vi "GetIPAddress.vi"() -> (0 "data out":string)   [LabVIEW 2012]
doc: "Get the RIO's IP address"
panel:
  out "error out":errorcluster
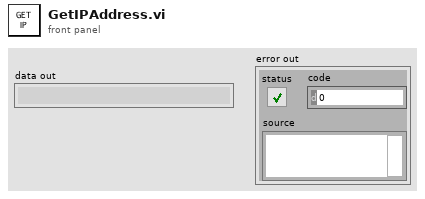
[diagram p1: front panel]
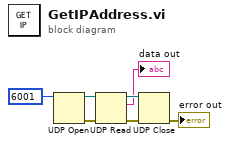
[diagram p0: block diagram]
diagram:
  n1 = UDP Open(11:u16 6001 ("port")) -> (port=w6:refnum<k16>, 0:w7:errorcluster)  [unwired: 4 in, 1 out]
  n2 = UDP Read(connection ID=w6, 8:w7) -> (data out=→"data out":string, error out=w4:errorcluster, 3:w3:refnum<k16>)  [unwired: 2 in, 2 out]
  n3 = UDP Close(connection ID=w3, 8:w4) -> (error out=→"error out":errorcluster)  [unwired: 1 out]
